vi "FPGA_DMAStopTransfer.vi"(8 "error in (no error)":errorcluster, 11 "DMADevRef In":T1) -> (0 "error out":errorcluster, 3 "DMADevRef Out":T1)   [LabVIEW 2017]
uses:
  <vilib>/Rock Robotics/SystemInterfaces/DMA/FPGA_DMADevRef.ctl
  <vilib>/Rock Robotics/SystemInterfaces/System/FPGA_SystemFPGA Ref Global.vi
  <vilib>/Utility/error.llb/Error Cluster From Error Code.vi
  <vilib>/rvi/interface/nirviMethod/nirviMethod.xnode
  <vilib>/Rock Robotics/SystemInterfaces/System/FPGA_SystemFRC FPGA Ref.ctl
  <vilib>/FPGAPlugInAG/Dynamic/niLvFpga_StopFifo_Dynamic.vi
  <vilib>/rvi/errors/niLvFpgaMergeErrorWithErrorCode.vi
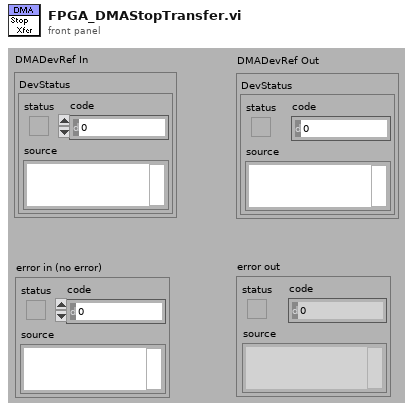
[diagram p1: front panel]
types:
  T1 = typedef "FPGA_DMADevRef.ctl" = cluster{"DevStatus":errorcluster}
  T2 = typedef "FPGA_SystemFRC FPGA Ref.ctl" = refnum<k20>
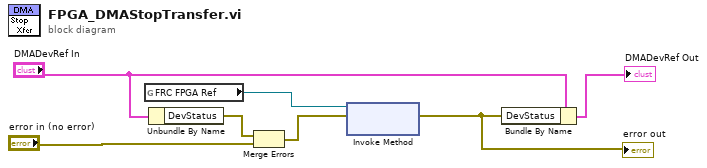
[diagram p0: block diagram]
diagram:
  n1 = global read "FPGA_SystemFPGA Ref Global.vi" "FRC FPGA Ref"() -> (w4:T2)
  n2 = Unbundle By Name("DMADevRef In") -> ("DevStatus"=w3:errorcluster)
  n3 = Merge Errors(w3, "error in (no error)") -> (w1:errorcluster)
  n4 = xnode "Invoke Method"("FPGA VI Reference In"=w4, "error in"=w1) -> ("error out"=w5:errorcluster)  [unwired: 1 out]
  "error out" <- w5
  n5 = Bundle By Name(cluster="DMADevRef In", "DevStatus"=w5) -> (→"DMADevRef Out":T1)
